vi "BundlePaths.vi"(0 "Data Path":path, 1 "UiDefinition 2":T1) -> (7 "UiDefinition 3":T1)   [LabVIEW 2020]
uses:
  UIReferences.ctl
  C:/Users/User/Desktop/Automation/CurrentVersion/LabviewDXFViewer/bin/Release/LabviewDXFViewer.exe
  LabviewDXFViewer/bin/Release/LabviewDXFViewer.exe
  <vilib>/wsapi/NI_WebServices.lvlib
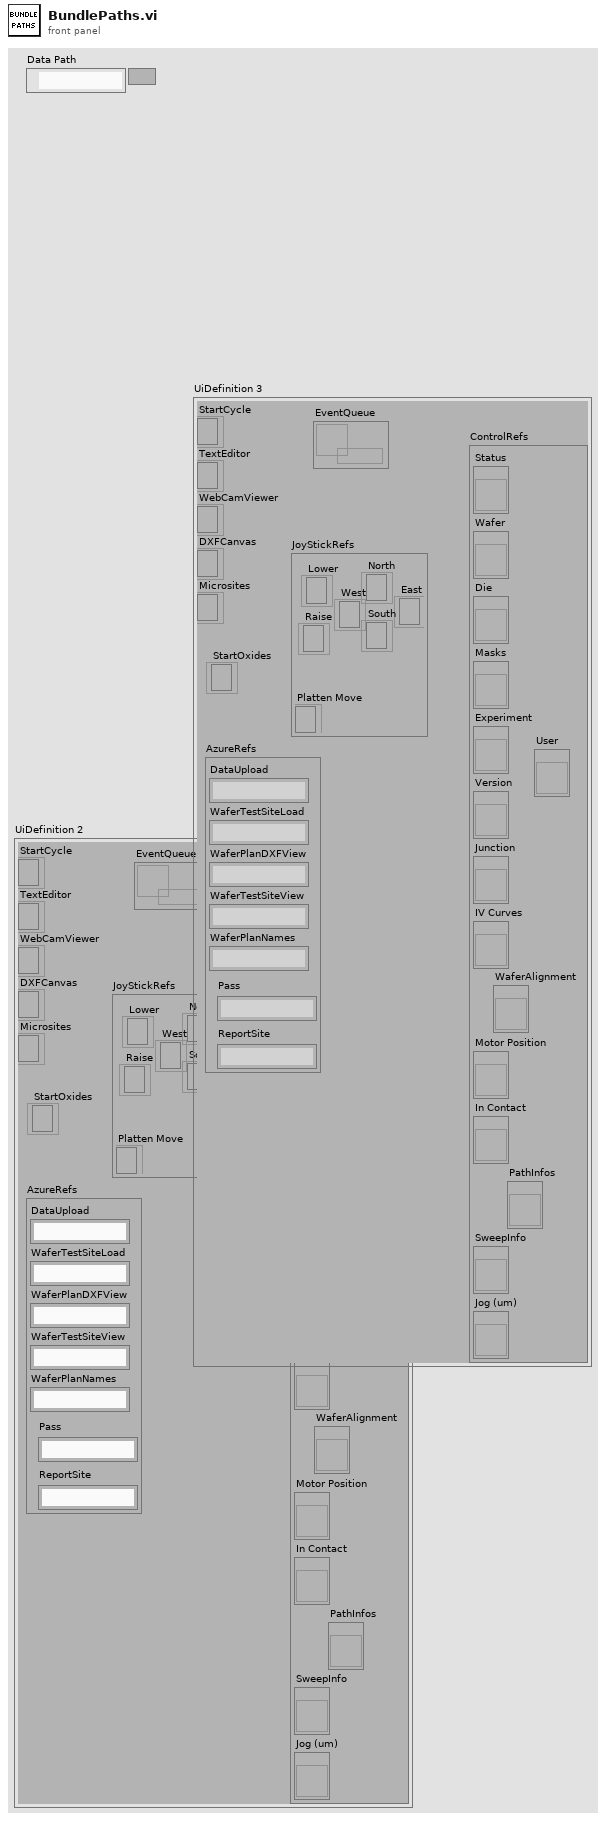
[diagram p1: front panel]
types:
  T1 = typedef "UIReferences.ctl" = cluster{"StartCycle":refnum<k24>, "TextEditor":refnum<k24>, "WebCamViewer":refnum<k24>, "DXFCanvas":refnum<k24>, "Microsites":refnum<k24>, "JoyStickRefs":cluster{"North":refnum<k24>, "Lower":refnum<k24>, "Raise":refnum<k24>, "Platten Move":refnum<k24>, "West":refnum<k24>, "East":refnum<k24>, "South":refnum<k24>}, "AzureRefs":cluster{"DataUpload":string, "WaferTestSiteLoad":string, "WaferPlanDXFView":string, "WaferTestSiteView":string, "WaferPlanNames":string, "Pass":string, "ReportSite":string}, "ControlRefs":cluster{"Status":refnum<vi>, "Wafer":refnum<vi>, "Die":refnum<vi>, "Masks":refnum<vi>, "Experiment":refnum<vi>, "Version":refnum<vi>, "Junction":refnum<vi>, "IV Curves":refnum<vi>, "Motor Position":refnum<vi>, "In Contact":refnum<vi>, "SweepInfo":refnum<vi>, "Jog (um)":refnum<vi>, "PathInfos":refnum<vi>, "User":refnum<vi>, "WaferAlignment":refnum<vi>}, "EventQueue":refnum<queue>, "StartOxides":refnum<k24>}
  T2 = cluster{"DataUpload":string, "WaferTestSiteLoad":string, "WaferPlanDXFView":string, "WaferTestSiteView":string, "WaferPlanNames":string, "Pass":string, "ReportSite":string}
  T3 = cluster{"Die":string, "Wafer":string, "Path":path, "url":string, "Experiment":string, "Version":string, "user":string}
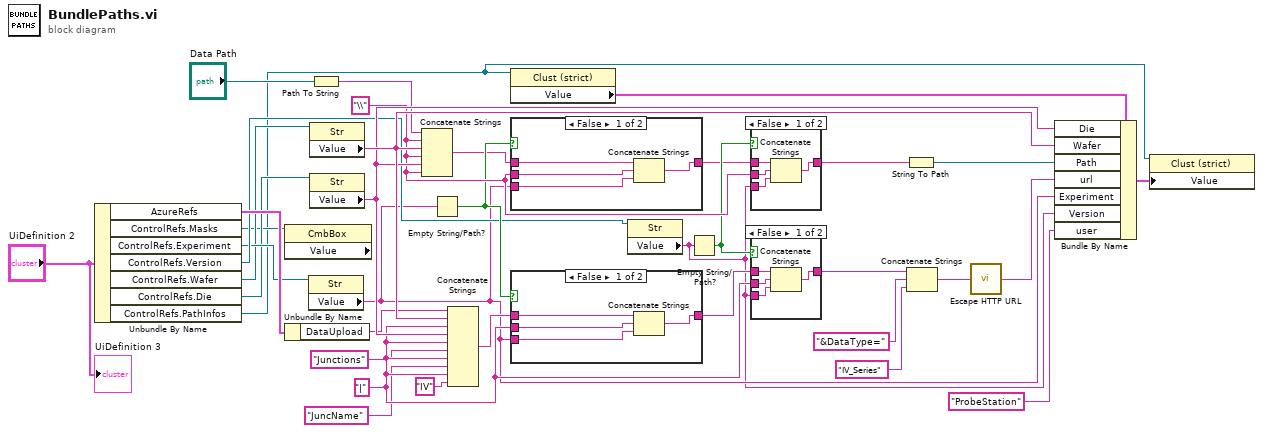
[diagram p0: block diagram]
diagram:
  w32 = "\\" ("string")
  w27 = "|" ("delimiter (\\t)")
  n1 = Unbundle By Name("UiDefinition 2") -> ("AzureRefs"=w12:T2, "ControlRefs.Masks"=w7:refnum<vi>, "ControlRefs.Experiment"=w10:refnum<vi>, "ControlRefs.Version"=w11:refnum<vi>, "ControlRefs.Wafer"=w9:refnum<vi>, "ControlRefs.Die"=w8:refnum<vi>, "ControlRefs.PathInfos"=w5:refnum<vi>)
  n2 = property class="CmbBox" props=["Value"](reference=w7) -> ()  [unwired: 1 in, 3 out]
  n3 = Unbundle By Name(w12) -> ("DataUpload"=w18:string)
  n4 = property class="Str"(reference=w10) -> ("Value"=w3:string)  [unwired: 1 in, 2 out]
  n5 = property class="Str"(reference=w9) -> ("Value"=w36:string)  [unwired: 1 in, 2 out]
  n6 = property class="Str"(reference=w8) -> ("Value"=w35:string)  [unwired: 1 in, 2 out]
  n7 = Path To String(path="Data Path") -> (string=w33:string)
  n8 = Concatenate Strings(w33, w32, w36, w32, w35, w32) -> (w15:string)
  n9 = Empty String/Path?(string/path=w3) -> (empty?=w22:bool)
  n10 = Concatenate Strings(w18, w36, w27, w35, w27, "Junctions" ("string"), w27, "JuncName" ("string"), w27, "IV" ("string")) -> (w21:string)
  n11 = property class="Clust (strict)"(reference=w5) -> ("Value"=w6:T3)  [unwired: 1 in, 2 out]
  n12 = case shown="False" w22 {
    tunnel: w15 -> [w40 w41]
    tunnel: [w38 w41] -> w16
    tunnel: w32 -> [w39 _]
    tunnel: w3 -> [w37 _]
    frame False {
      n13 = Concatenate Strings(w40, w39, w37) -> (w38:string)
    }
    frame True {
    }
  }
  n14 = case shown="False" w22 {
    tunnel: w21 -> [w45 w46]
    tunnel: w3 -> [w43 _]
    tunnel: [w44 w46] -> w23
    tunnel: w27 -> [w42 _]
    frame False {
      n15 = Concatenate Strings(w45, w42, w43) -> (w44:string)
    }
    frame True {
    }
  }
  n16 = property class="Str"(reference=w11) -> ("Value"=w2:string)  [unwired: 1 in, 2 out]
  n17 = Empty String/Path?(string/path=w2) -> (empty?=w31:bool)
  n18 = case shown="False" w31 {
    tunnel: [w50 w51] -> w17
    tunnel: w16 -> [w49 w51]
    tunnel: w32 -> [w48 _]
    tunnel: w2 -> [w47 _]
    frame False {
      n19 = Concatenate Strings(w49, w48, w47) -> (w50:string)
    }
    frame True {
    }
  }
  n20 = case shown="False" w31 {
    tunnel: w23 -> [w55 w56]
    tunnel: [w52 w56] -> w24
    tunnel: w27 -> [w54 _]
    tunnel: w2 -> [w53 _]
    frame False {
      n21 = Concatenate Strings(w55, w54, w53) -> (w52:string)
    }
    frame True {
    }
  }
  n22 = String To Path(string=w17) -> (path=w34:path)
  n23 = Concatenate Strings(w24, "&DataType=" ("string"), "IV_Series" ("string")) -> (w25:string)
  n24 = call <vilib>:"Escape HTTP URL.vi"("unescaped string in"=w25) -> ("escaped string out"=w20:string)
  n25 = Bundle By Name(cluster=w6, "Die"=w35, "Wafer"=w36, "Path"=w34, "url"=w20, "Experiment"=w3, "Version"=w2, "user"="ProbeStation") -> (w4:T3)
  n26 = property class="Clust (strict)"(reference=w5, "Value"=w4) -> ()  [unwired: 1 in, 2 out]
  "UiDefinition 3" <- "UiDefinition 2"
